vi "svfa_No Average Array (complex).vi"(0 "array":cdb[](array[numeric]) format="%.2f", 11 "error in (no error)":errorcluster) -> (4 "dup array":cdb[](array[numeric]) format="%.2f", 6 "new spectrum ready":bool, 8 "averaging done":bool, 10 "averages completed":dbl, 15 "error out":errorcluster)   [LabVIEW 2017]
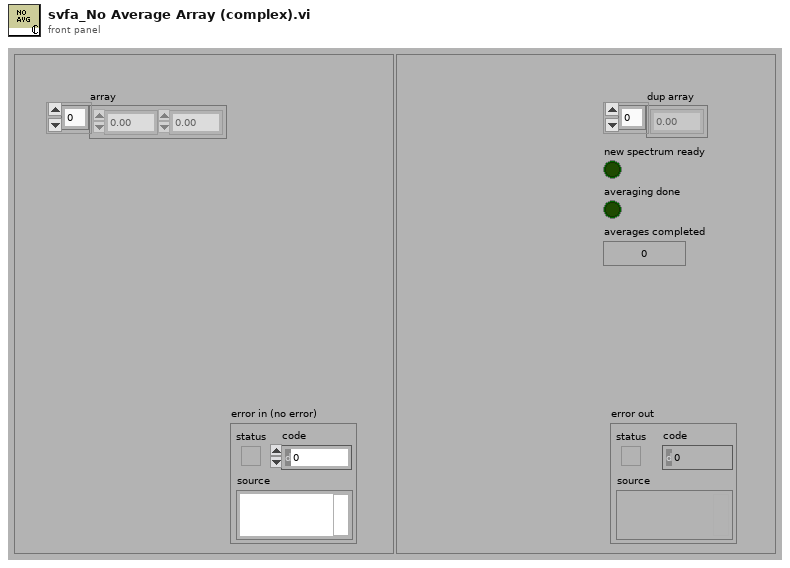
[diagram p1: front panel]
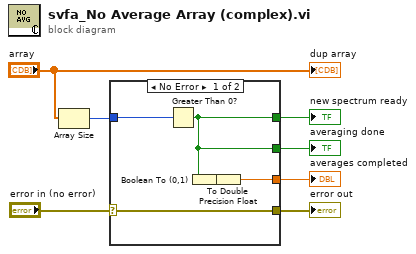
[diagram p0: block diagram]
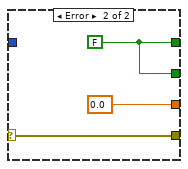
[diagram p2: hidden frame]
diagram:
  n1 = Array Size(array="array") -> (size(s)=w1:i32)
  n2 = case shown="No Error" "error in (no error)" {
    selector: "error in (no error)" -> [w10 w15]
    tunnel: [w11 0.0] -> w7
    tunnel: [w12 w14] -> w6
    tunnel: [w12 w14] -> w5
    tunnel: [w10 w15] -> w3
    tunnel: w1 -> [w8 _]
    frame No Error {
      n3 = Greater Than 0?(x=w8) -> (x > 0?=w12:bool)
      n4 = Boolean To (0,1)(Boolean=w12) -> (0, 1=w9:i16)
      n5 = To Double Precision Float(number=w9) -> (double precision float=w11:dbl)
    }
    frame Error {
      w14 = FALSE
    }
  }
  "averages completed" <- w7
  "new spectrum ready" <- w6
  "averaging done" <- w5
  "error out" <- w3
  "dup array" <- "array"
